vi "Facade.vi"(0 "Data In":T7, 2 "Display State In":T2={"Draw Options"={"Background Color"=16777215, "Grid Color"=13816530, "Angle Units"=enum."Radians", "Draw Solid Background"=TRUE, "Draw Grid"=TRUE, "Grid Spacing"=1.0, "AutoScale"=TRUE, "Fit to Radius"=1.0, "data row options"=[]}}, 3 "Container State":T6) -> (6 "Data Out":T7, 7 "Display State Out":T2={"Draw Options"={"Background Color"=16777215, "Grid Color"=13816530, "Angle Units"=enum."Radians", "Draw Solid Background"=TRUE, "Draw Grid"=TRUE, "Grid Spacing"=1.0, "AutoScale"=TRUE, "Fit to Radius"=1.0, "data row options"=[]}}, 8 "Action":T1)   [LabVIEW 2017, in "NI_Robotics_2D Rangefinder.xctl"]
uses:
  <vilib>/robotics/Controls/2D Rangefinder/NI_Robotics_2D Rangefinder.xctl
  <vilib>/robotics/Controls/2D Rangefinder/_2D Rangefinder Support Files/Data.ctl
  <vilib>/_xctls/Container State.ctl
  <vilib>/robotics/Controls/2D Rangefinder/_2D Rangefinder Support Files/State.ctl
  <vilib>/robotics/Controls/2D Rangefinder/2D Rangefinder Picture/Draw Options.ctl
  <vilib>/robotics/Controls/Utilities/Angle Units.ctl
  <vilib>/robotics/Controls/2D Rangefinder/2D Rangefinder Picture/Data Row Options.ctl
  <vilib>/_xctls/Action.ctl
  <vilib>/_xctls/XControlSupport.lvlib
  <vilib>/robotics/Controls/Utilities/NI_Robotics_Control Utilities.lvlib
  <vilib>/robotics/Controls/2D Rangefinder/_2D Rangefinder Support Files/Configuration/Config Dialog.lvlib
  <vilib>/robotics/Controls/2D Rangefinder/2D Rangefinder Picture/NI_Robotics_2D Rangefinder Picture.lvlib
panel:
  out "2D Picture":picture
types:
  T1 = typedef "XControlSupport.lvlib/Action.ctl" = cluster{"Data Changed?":bool, "State Changed?":bool, "Action Name":string}
  T2 = typedef "NI_Robotics_2D Rangefinder.xctl/State.ctl" = cluster{"Draw Options":T3}
  T3 = typedef "NI_Robotics_2D Rangefinder Picture.lvlib/Draw Options.ctl" = cluster{"Background Color":u32, "Grid Color":u32, "Angle Units":T4, "Draw Solid Background":bool, "Draw Grid":bool, "Grid Spacing":dbl, "AutoScale":bool, "Fit to Radius":dbl, "data row options":T5[]}
  T4 = typedef "NI_Robotics_Control Utilities.lvlib/Angle Units.ctl" = enum16{"Radians", "Degrees"}
  T5 = typedef "NI_Robotics_2D Rangefinder Picture.lvlib/Data Row Options.ctl" = cluster{"point color":u32, "line color":u32, "draw points":bool, "draw lines":bool, "point pixel size":u16, "max line distance":dbl, "line pixel width":u16}
  T6 = typedef "XControlSupport.lvlib/Container State.ctl" = cluster{"Indicator?":bool, "Run Mode?":bool, " Refnum":refnum<vi>}
  T7 = typedef "NI_Robotics_2D Rangefinder.xctl/Data.ctl" = cluster{"angle":dbl[], "distance":dbl[][]}
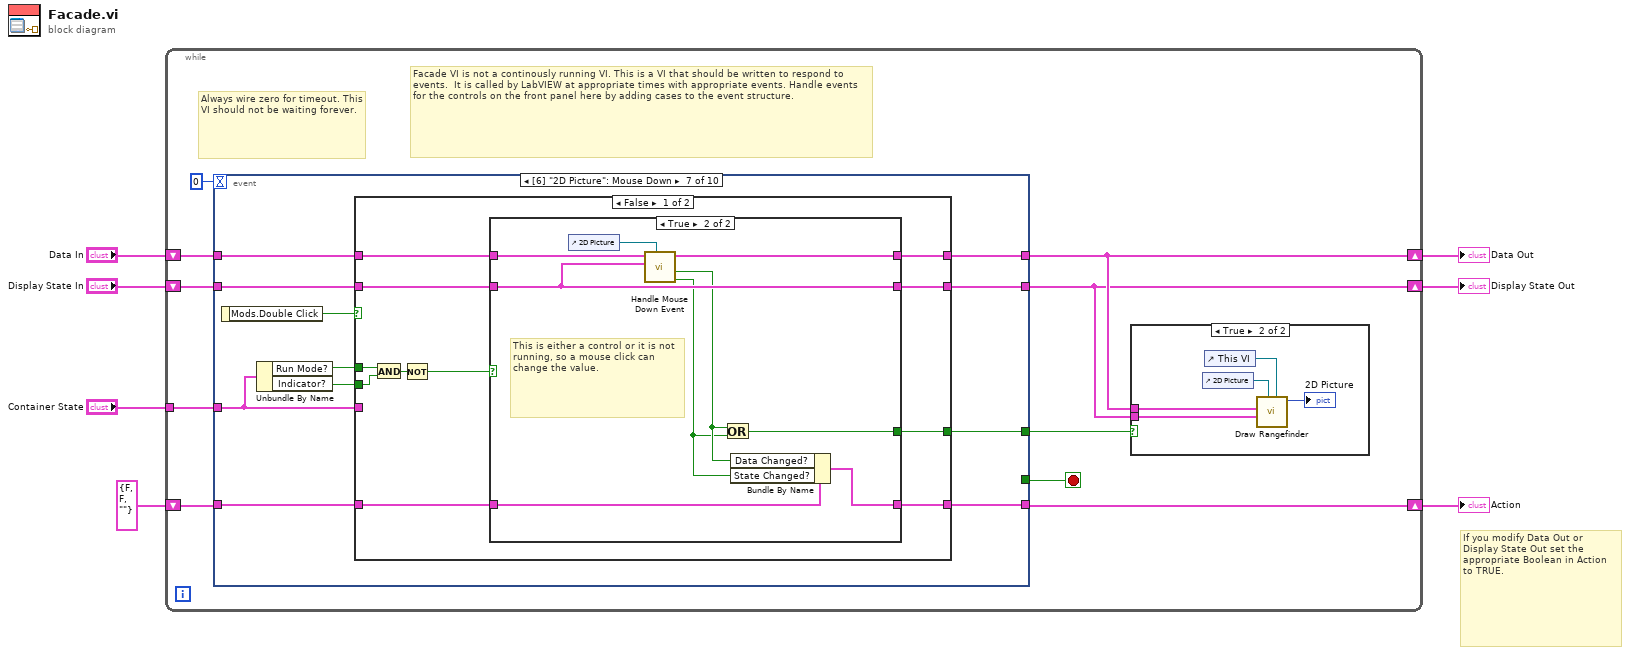
[diagram p0: block diagram]
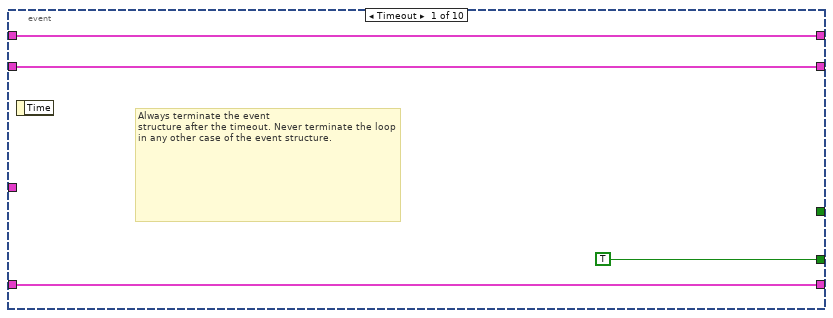
[diagram p3: hidden frame]
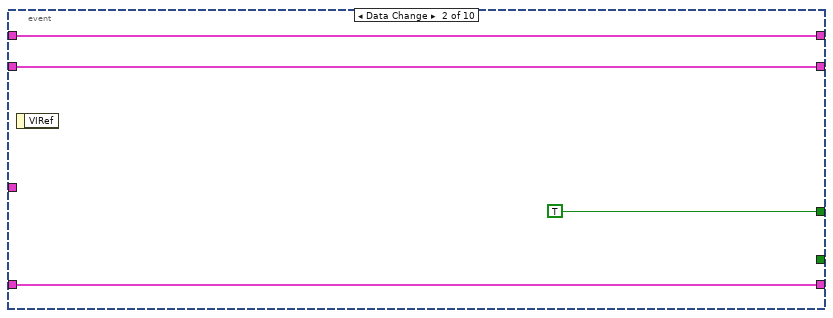
[diagram p4: hidden frame]
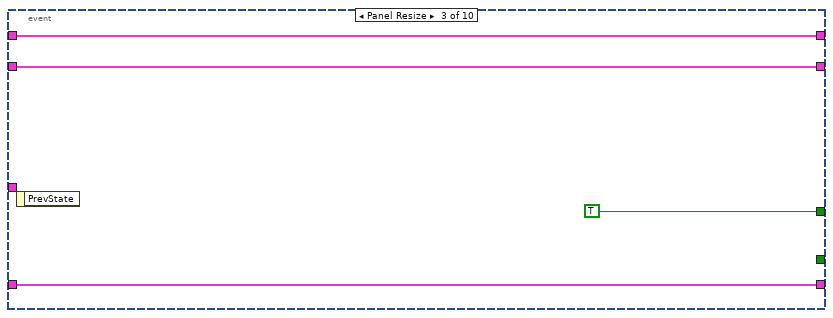
[diagram p5: hidden frame]
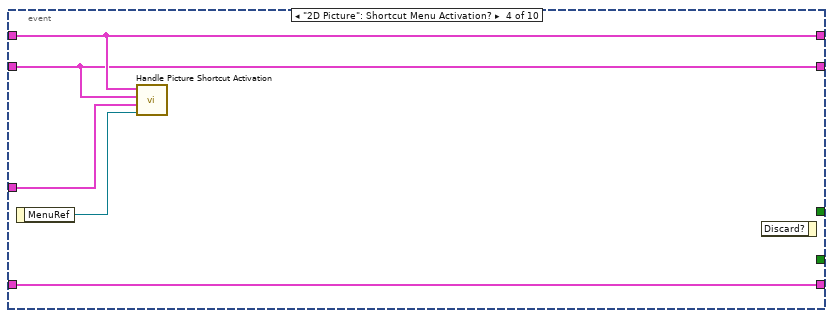
[diagram p6: hidden frame]
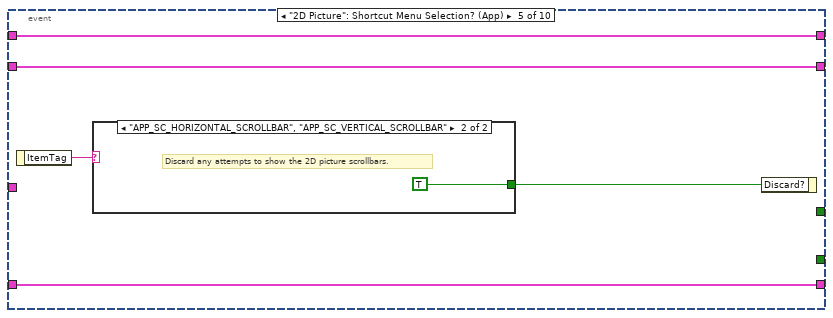
[diagram p7: hidden frame]
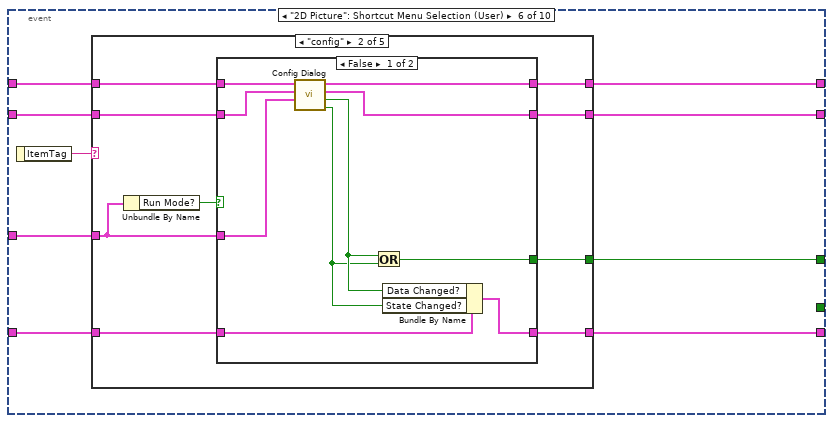
[diagram p9: hidden frame]
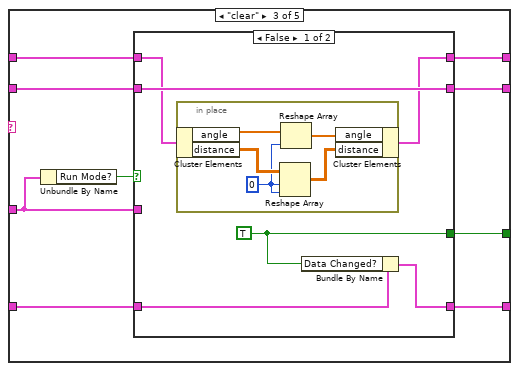
[diagram p12: hidden frame]
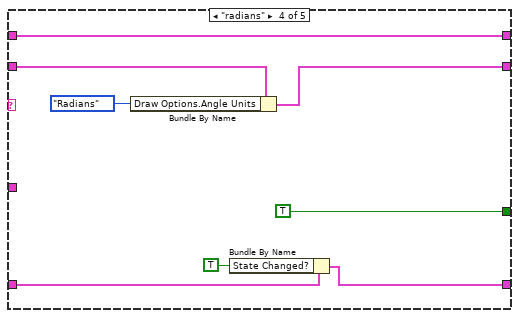
[diagram p14: hidden frame]
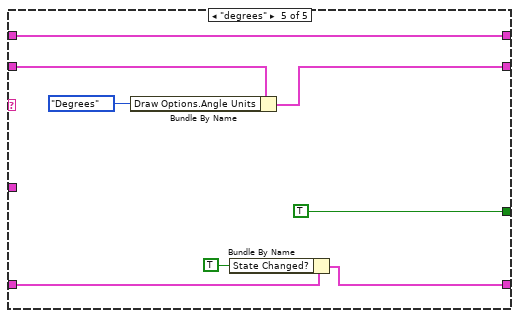
[diagram p15: hidden frame]
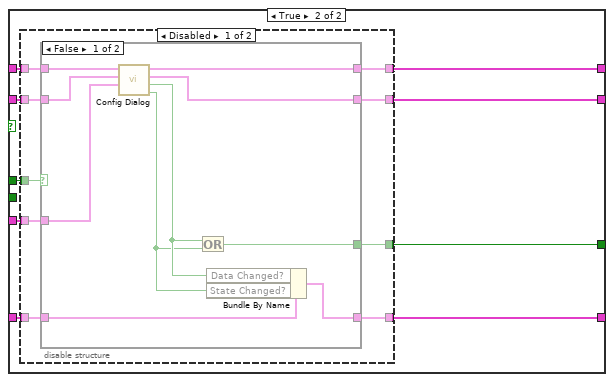
[diagram p17: hidden frame]
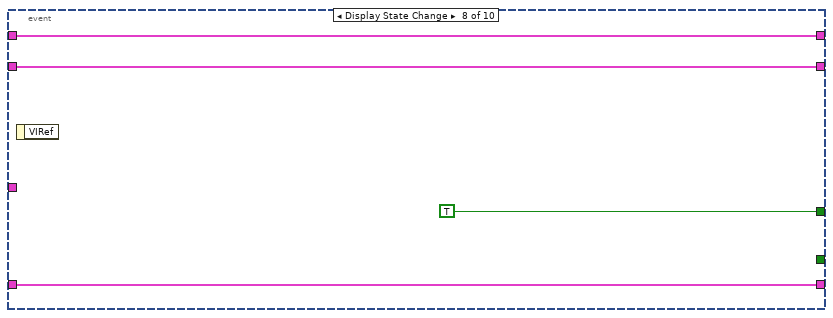
[diagram p20: hidden frame]
diagram:
  # "If you modify Data Out or\nDisplay State Out set the\nappropriate Boolean in Action\nto TRUE."
  n1 = while {
    shift-right: [w8] -> w1
    shift-left: "Display State In" -> [w17]
    tunnel: "Container State" -> [w14]
    shift-right: [w9] -> w7
    shift-left: "Data In" -> [w13]
    shift-right: [w11] -> w3
    shift-left: T1 {"Data Changed?"=FALSE, "State Changed?"=FALSE, "Action Name"=""} ("Action") -> [w12]
    stop <- w16 stop-if-true
    # "Facade VI is not a continously running VI. This is a VI that should be written to respond to events.  It is called by LabVIEW at appropriate times with appropriate events. Handle events for the controls on the front panel here by adding cases to the event structure."
    # "Always wire zero for timeout. This\nVI should not be waiting forever."
    n2 = event shown="[6] \"2D Picture\": Mouse Down" {
      selector: _ -> [_ _ _ _ _ _ _ _ _ _]
      dyn-events: _ -> [_ _ _ _ _ _ _ _ _ _]
      timeout: 0 -> [_ _ _ _ _ _ _ _ _ _]
      tunnel: w17 -> [w24 w29 w32 w35 w44 w53 w125 w188 w193 w196]
      tunnel: [w24 w29 w32 w35 w44 w52 w126 w188 w193 w196] -> w8
      tunnel: [TRUE _ _ _ _ _ _ _ _ _] -> w16
      tunnel: w14 -> [_ _ _ w37 _ w51 w121 _ _ _]
      tunnel: w13 -> [w23 w30 w33 w36 w43 w47 w129 w190 w192 w195]
      tunnel: [w23 w30 w33 w36 w43 w46 w127 w190 w192 w195] -> w9
      tunnel: [w25 w28 w31 w39 w42 w48 w123 w189 w191 w194] -> w11
      tunnel: w12 -> [w25 w28 w31 w39 w42 w49 w122 w189 w191 w194]
      tunnel: [_ TRUE TRUE _ _ w50 w124 TRUE _ _] -> w10
      event Timeout {
        # "Always terminate the event\nstructure after the timeout. Never terminate the loop in any other case of the event structure."
        n3 = event-data() -> ()  [unwired: 1 in, 1 out]
      }
      event Data Change {
        n4 = event-data() -> ()  [unwired: 1 in, 1 out]
      }
      event Panel Resize {
        n5 = event-data() -> ()  [unwired: 1 in, 1 out]
      }
      event "2D Picture": Shortcut Menu Activation? {
        n6 = event-data() -> ("MenuRef"=w38:refnum<k9>)  [unwired: 1 in]
        n7 = call <vilib>:"Handle Picture Shortcut Activation.vi"("MenuRef"=w38, "Container State"=w37, "state in"=w35, "data in"=w36) -> ()  [unwired: 8 in]
        n8 = event-data() -> ()  [unwired: 2 in, 1 out]
      }
      event "2D Picture": Shortcut Menu Selection? (App) {
        n9 = event-data() -> ("ItemTag"=w41:string)  [unwired: 1 in]
        n10 = case shown="\"APP_SC_HORIZONTAL_SCROLLBAR\", \"APP_SC_VERTICAL_SCROLLBAR\"" w41 {
          tunnel: [_ TRUE] -> w40
          frame Default {
          }
          frame "APP_SC_HORIZONTAL_SCROLLBAR", "APP_SC_VERTICAL_SCROLLBAR" {
            # "Discard any attempts to show the 2D picture scrollbars."
          }
        }
        n11 = event-data("Discard?"=w40) -> ()  [unwired: 1 in, 1 out]
      }
      event "2D Picture": Shortcut Menu Selection (User) {
        n12 = event-data() -> ("ItemTag"=w54:string)  [unwired: 1 in]
        n13 = case shown="\"config\"" w54 {
          tunnel: w53 -> [w57 w65 w87 w109 w117]
          tunnel: [w57 w66 w88 w108 w116] -> w52
          tunnel: w51 -> [_ w58 w80 _ _]
          tunnel: [_ w64 w86 TRUE TRUE] -> w50
          tunnel: w49 -> [w56 w62 w84 w107 w115]
          tunnel: [w56 w61 w83 w106 w114] -> w48
          tunnel: w47 -> [w55 w60 w82 w110 w118]
          tunnel: [w55 w59 w81 w110 w118] -> w46
          frame Default {
          }
          frame "config" {
            n14 = Unbundle By Name(w58) -> ("Run Mode?"=w63:bool)
            n15 = case shown="False" w63 {
              tunnel: w65 -> [w72 w79]
              tunnel: [w70 w79] -> w66
              tunnel: [w67 _] -> w64
              tunnel: w62 -> [w76 w77]
              tunnel: [w75 w77] -> w61
              tunnel: w60 -> [w74 w78]
              tunnel: [w73 w78] -> w59
              tunnel: w58 -> [w71 _]
              frame False {
                n16 = call <vilib>:"Config Dialog.vi"("Container State"=w71, "state in"=w72, "data in"=w74) -> ("state changed?"=w68:bool, "data changed?"=w69:bool, "state out"=w70:T2, "data out"=w73:T7)  [unwired: 5 in]
                n17 = Or(x=w69, y=w68) -> (x .or. y?=w67:bool)
                n18 = Bundle By Name(cluster=w76, "Data Changed?"=w69, "State Changed?"=w68) -> (w75:T1)
              }
              frame True {
              }
            }
          }
          frame "clear" {
            n19 = Unbundle By Name(w80) -> ("Run Mode?"=w85:bool)
            n20 = case shown="False" w85 {
              tunnel: w87 -> [w92 w102]
              tunnel: [w92 w102] -> w88
              tunnel: [w91 _] -> w86
              tunnel: w84 -> [w94 w100]
              tunnel: [w93 w100] -> w83
              tunnel: w82 -> [w90 w101]
              tunnel: [w89 w101] -> w81
              tunnel: w80 -> [_ _]
              frame False {
                w91 = TRUE
                n21 = in-place {
                  w95 = 0 ("dimension size")
                  n22 = in-place-cluster #1(w90) -> ("angle"=w99:dbl[], "distance"=w97:dbl[][])
                  n23 = Reshape Array(w97, w95, w95) -> (w96:dbl[][])
                  n24 = Reshape Array(w99, w95) -> (w98:dbl[])
                  n25 = in-place-cluster #1("angle"=w98, "distance"=w96) -> (w89:T7)
                }
                n26 = Bundle By Name(cluster=w94, "Data Changed?"=w91) -> (w93:T1)
              }
              frame True {
              }
            }
          }
          frame "radians" {
            n27 = Bundle By Name(cluster=w109, "Draw Options.Angle Units"=Angle_Units."Radians") -> (w108:T2)
            n28 = Bundle By Name(cluster=w107, "State Changed?"=TRUE) -> (w106:T1)
          }
          frame "degrees" {
            n29 = Bundle By Name(cluster=w117, "Draw Options.Angle Units"=Angle_Units."Degrees") -> (w116:T2)
            n30 = Bundle By Name(cluster=w115, "State Changed?"=TRUE) -> (w114:T1)
          }
        }
      }
      event "2D Picture": Mouse Down {
        n31 = event-data() -> ("Mods.Double Click"=w128:bool)  [unwired: 1 in]
        n32 = Unbundle By Name(w121) -> ("Run Mode?"=w120:bool, "Indicator?"=w119:bool)
        n33 = case shown="False" w128 {
          tunnel: w125 -> [w135 w160]
          tunnel: [w134 w161] -> w126
          tunnel: w121 -> [_ w154]
          tunnel: [w131 w159] -> w124
          tunnel: w122 -> [w133 w158]
          tunnel: [w132 w157] -> w123
          tunnel: w129 -> [w137 w156]
          tunnel: [w136 w155] -> w127
          tunnel: w120 -> [w140 w153]
          tunnel: w119 -> [w139 _]
          frame False {
            n34 = And(x=w140, y=w139) -> (x .and. y?=w138:bool)
            n35 = Not(x=w138) -> (.not. x?=w130:bool)
            n36 = case shown="True" w130 {
              tunnel: w137 -> [w143 w152]
              tunnel: [w143 w151] -> w136
              tunnel: w135 -> [w142 w147]
              tunnel: [w142 w147] -> w134
              tunnel: w133 -> [w141 w149]
              tunnel: [w141 w148] -> w132
              tunnel: [_ w144] -> w131
              frame False {
              }
              frame True {
                # "This is either a control or it is not running, so a mouse click can  change the value."
                n37 = control-ref of="2D Picture"() -> (w150:refnum<vi>)
                n38 = call <vilib>:"Handle Mouse Down Event.vi"("2D Picture"=w150, "state in"=w147, "data in"=w152) -> ("state changed?"=w145:bool, "data changed?"=w146:bool, "data out"=w151:T7)  [unwired: 6 in]
                n39 = Or(x=w146, y=w145) -> (x .or. y?=w144:bool)
                n40 = Bundle By Name(cluster=w149, "Data Changed?"=w146, "State Changed?"=w145) -> (w148:T1)
              }
            }
          }
          frame True {
            n41 = disable-structure shown="Disabled" {
              disable-tunnel: [w170 w185] -> w161
              disable-tunnel: w160 -> [w169 w185]
              disable-tunnel: [w168 _] -> w159
              disable-tunnel: w158 -> [w167 w184]
              disable-tunnel: [w166 w184] -> w157
              disable-tunnel: w156 -> [w165 w186]
              disable-tunnel: [w164 w186] -> w155
              disable-tunnel: w154 -> [w163 _]
              disable-tunnel: w153 -> [w162 _]
              frame Disabled {
                n42 = case shown="False" w162 {
                  tunnel: w169 -> [w176 w183]
                  tunnel: [w174 w183] -> w170
                  tunnel: [w171 _] -> w168
                  tunnel: w167 -> [w180 w181]
                  tunnel: [w179 w181] -> w166
                  tunnel: w165 -> [w178 w182]
                  tunnel: [w177 w182] -> w164
                  tunnel: w163 -> [w175 _]
                  frame False {
                    n43 = call <vilib>:"Config Dialog.vi"("Container State"=w175, "state in"=w176, "data in"=w178) -> ("state changed?"=w172:bool, "data changed?"=w173:bool, "state out"=w174:T2, "data out"=w177:T7)  [unwired: 5 in]
                    n44 = Or(x=w173, y=w172) -> (x .or. y?=w171:bool)
                    n45 = Bundle By Name(cluster=w180, "Data Changed?"=w173, "State Changed?"=w172) -> (w179:T1)
                  }
                  frame True {
                  }
                }
              }
              frame Enabled {
              }
            }
          }
        }
      }
      event Display State Change {
        n46 = event-data() -> ()  [unwired: 1 in, 1 out]
      }
      event Direction Change {
        n47 = event-data() -> ()  [unwired: 1 in, 1 out]
      }
      event Exec State Change {
        n48 = event-data() -> ()  [unwired: 1 in, 1 out]
      }
    }
    n49 = case shown="True" w10 {
      tunnel: w9 -> [_ w20]
      tunnel: w8 -> [_ w18]
      frame False {
      }
      frame True {
        n50 = control-ref of="2D Picture"() -> (w21:refnum<vi>)
        n51 = control-ref of="This VI"() -> (w22:refnum<vi>)
        n52 = call <vilib>:"Draw Rangefinder.vi"("FcdVI Refnum"=w22, "2D Picture"=w21, "State"=w18, "data"=w20) -> ("Picture Out"=→"2D Picture":picture)  [unwired: 7 in]
      }
    }
  }
  "Display State Out" <- w1
  "Data Out" <- w7
  "Action" <- w3
